vi "PRBS.vi"(7 "Fréquence \nd'echantillonage (Hz)":dbl, 8 "Entrée d'erreur\n(sans erreur)":errorcluster caption="Error in (no error)", 11 "Labview opt":T1={"Fréequence minimale (Hz)"=0.1, "Amplitude minimale (V)"=0.0, "Amplitude maximale (V)"=1.0, "Fréquence maximale (Hz)"=0.1, "Temps de simulation (min)"=2.0}) -> (0 "Sorti d'erreur":errorcluster, 2 "DSP par FFT":cluster{dbl[], dbl[]}(graph) caption="DSP approximée", 3 "u":cluster{dbl[], dbl[]}(graph))   [LabVIEW 2019]
uses:
  <vilib>/Analysis/NI_AALPro.lvlib
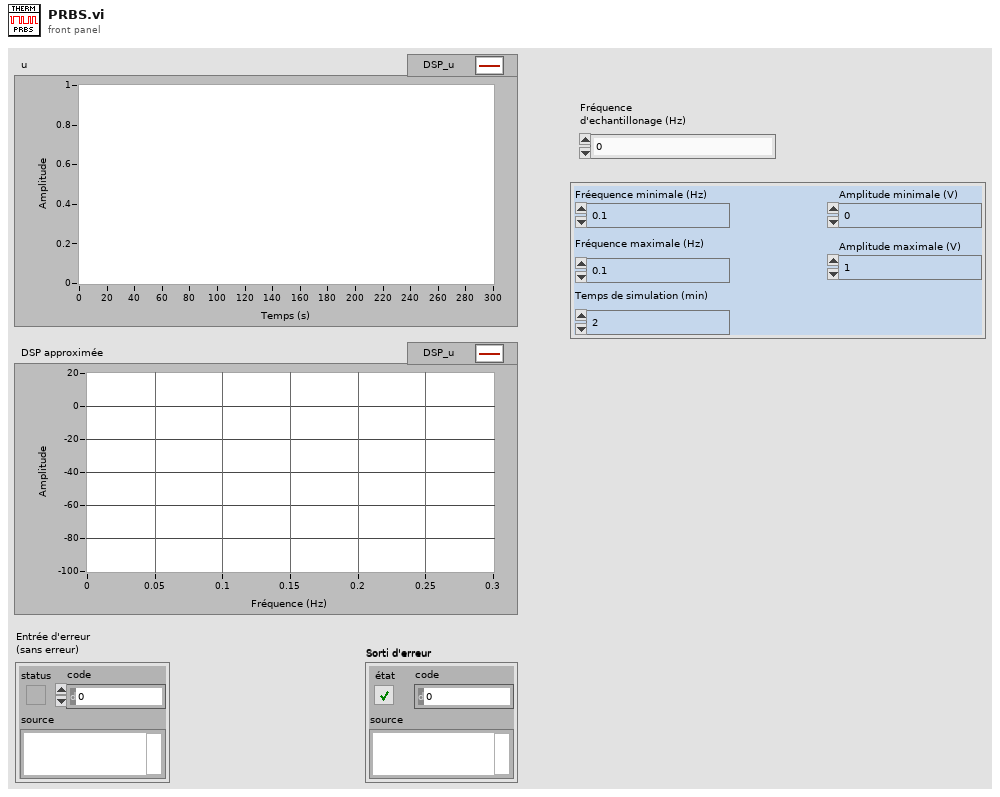
[diagram p1: front panel]
types:
  T1 = cluster{"Fréequence minimale (Hz)":dbl, "Amplitude minimale (V)":dbl, "Amplitude maximale (V)":dbl, "Fréquence maximale (Hz)":dbl, "Temps de simulation (min)":dbl}
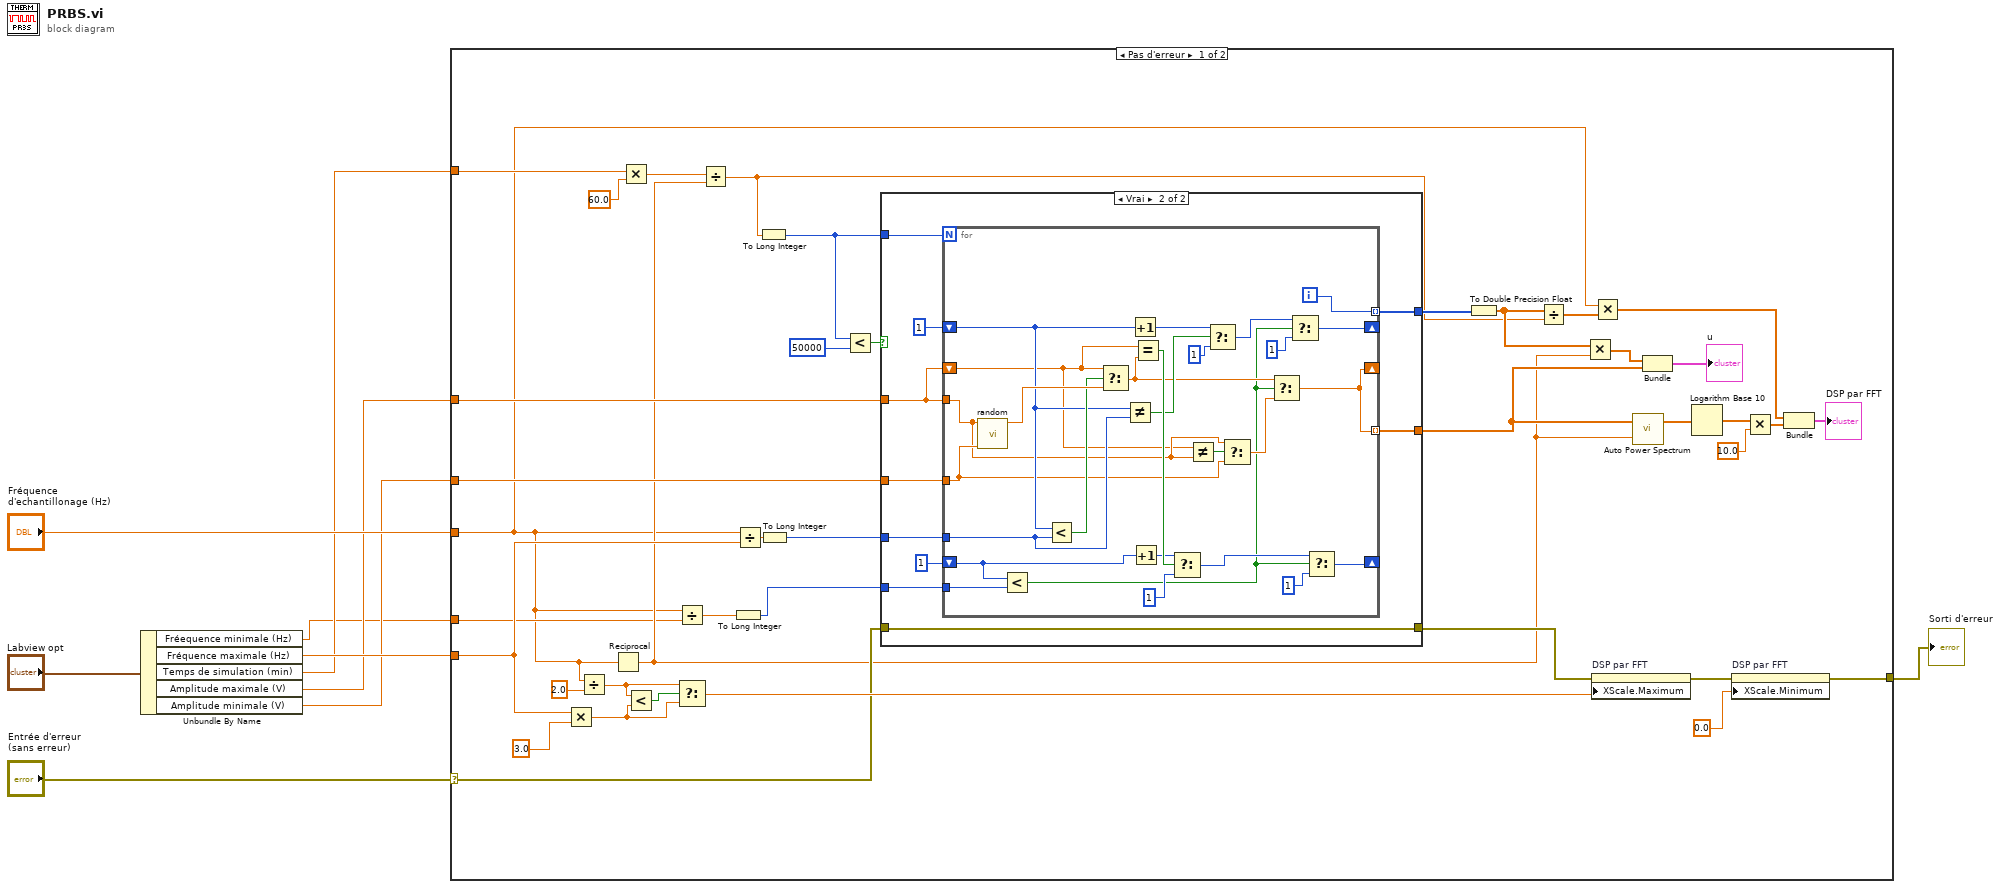
[diagram p0: block diagram]
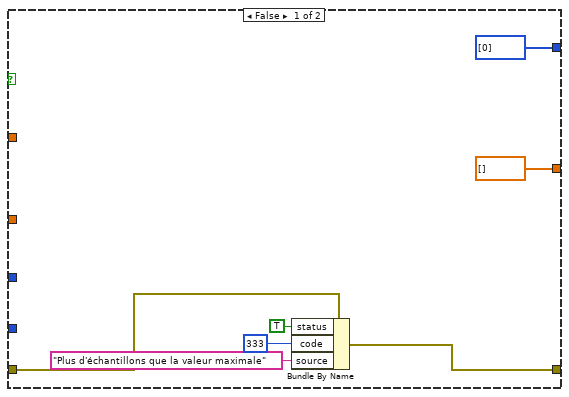
[diagram p2: hidden frame]
diagram:
  n1 = Unbundle By Name("Labview opt") -> ("Fréequence minimale (Hz)"=w1:dbl, "Fréquence maximale (Hz)"=w6:dbl, "Temps de simulation (min)"=w5:dbl, "Amplitude maximale (V)"=w3:dbl, "Amplitude minimale (V)"=w4:dbl)
  n2 = case shown="Pas d'erreur" "Entrée d'erreur\n(sans erreur)" {
    selector: "Entrée d'erreur\n(sans erreur)" -> [w16 w94]
    tunnel: "Fréquence \nd'echantillonage (Hz)" -> [w10 _]
    tunnel: w6 -> [w35 _]
    tunnel: [w27 w94] -> w7
    tunnel: w5 -> [w23 _]
    tunnel: w4 -> [w22 _]
    tunnel: w3 -> [w21 _]
    tunnel: w1 -> [w11 _]
    frame No Error {
      n3 = Multiply(x=w35, y=3.0) -> (x*y=w34:dbl)
      n4 = Divide(x=w10, y=2.0) -> (x/y=w31:dbl)
      n5 = Reciprocal(x=w10) -> (1/x=w12:dbl)
      n6 = Multiply(x=w23, y=60.0) -> (x*y=w25:dbl)
      n7 = Less?(x=w31, y=w34) -> (x < y?=w33:bool)
      n8 = Divide(x=w10, y=w11) -> (x/y=w15:dbl)
      n9 = Select(t=w31, s=w33, f=w34) -> (s? t:f=w32:dbl)
      n10 = Divide(x=w25, y=w12) -> (x/y=w29:dbl)
      n11 = To Long Integer(number=w15) -> (32bit integer=w14:i32)
      n12 = Divide(x=w10, y=w35) -> (x/y=w49:dbl)
      n13 = To Long Integer(number=w29) -> (32bit integer=w20:i32)
      n14 = To Long Integer(number=w49) -> (32bit integer=w48:i32)
      n15 = Less?(x=w20, y=50000) -> (x < y?=w19:bool)
      n16 = case shown="Vrai" w19 {
        tunnel: w48 -> [_ w66]
        tunnel: [i32[] [0] w62] -> w41
        tunnel: [dbl[] [] w59] -> w13
        tunnel: w20 -> [_ w65]
        tunnel: w22 -> [_ w64]
        tunnel: w21 -> [_ w58]
        tunnel: [w50 w63] -> w17
        tunnel: w16 -> [w54 w63]
        tunnel: w14 -> [_ w60]
        frame False {
          n17 = Bundle By Name(cluster=w54, "status"=TRUE, "code"=333, "source"="Plus d'échantillons que la valeur maximale") -> (w50:errorcluster)
        }
        frame True {
          n18 = for {
            N: w65 -> [_]
            shift-right: [w69] -> _
            shift-left: w58 -> [w67]
            tunnel: w66 -> [w77]
            tunnel: w64 -> [w74]
            tunnel: w58 -> [w71]
            shift-right: [w89] -> _
            shift-left: 1 -> [w78]
            tunnel: [w93] -> w62 mode=indexing
            tunnel: w60 -> [w90]
            tunnel: [w69] -> w59 mode=indexing
            shift-right: [w82] -> _
            shift-left: 1 -> [w75]
            i -> [w93]
            n19 = call "random.vi"("Min value"=w74, "Max value"=w71) -> ("Sortie"=w80:dbl)  [unwired: 8 in, 1 out]
            n20 = Less?(x=w75, y=w90) -> (x < y?=w68:bool)
            n21 = Less?(x=w78, y=w77) -> (x < y?=w79:bool)
            n22 = Select(t=w67, s=w79, f=w80) -> (s? t:f=w72:dbl)
            n23 = Not Equal?(x=w78, y=w77) -> (x != y?=w76:bool)
            n24 = Increment(x=w78) -> (x+1=w92:i32)
            n25 = Increment(x=w75) -> (x+1=w84:i32)
            n26 = Equal?(x=w67, y=w72) -> (x = y?=w85:bool)
            n27 = Select(t=w84, s=w85, f=1 ("cas faux")) -> (s? t:f=w81:i32)
            n28 = Not Equal?(x=w67, y=w71) -> (x != y?=w70:bool)
            n29 = Select(t=w92, s=w76, f=1 ("cas faux")) -> (s? t:f=w88:i32)
            n30 = Select(t=w71, s=w70, f=w74) -> (s? t:f=w73:dbl)
            n31 = Select(t=w72, s=w68, f=w73) -> (s? t:f=w69:dbl)
            n32 = Select(t=w88, s=w68, f=1 ("cas faux")) -> (s? t:f=w89:i32)
            n33 = Select(t=w81, s=w68, f=1 ("cas faux")) -> (s? t:f=w82:i32)
          }
        }
      }
      n34 = To Double Precision Float(number=w41) -> (double precision float=w36:dbl[])
      n35 = Divide(x=w36, y=w29) -> (x/y=w40:dbl[])
      n36 = Multiply(x=w36, y=w12) -> (x*y=w37:dbl[])
      n37 = property on="DSP par FFT" class="GraphXY (strict)"(error in=w17, "XScale.Maximum"=w32) -> (error out=w28:errorcluster)  [unwired: 1 in, 1 out]
      n38 = Multiply(x=w10, y=w40) -> (x*y=w39:dbl[])
      n39 = call <vilib>:"Auto Power Spectrum.vi"("dt"=w12, "Signal (V)"=w13) -> ("Power Spectrum (V^2 rms)"=w47:dbl[])  [unwired: 1 out]
      n40 = Bundle(w37, w13) -> (→"u":cluster{dbl[], dbl[]})  [unwired: 1 in]
      n41 = Logarithm Base 10(1:w47) -> (0:w46:dbl[])
      n42 = property on="DSP par FFT" class="GraphXY (strict)"(error in=w28, "XScale.Minimum"=0.0 ("Échelle des X.Gamme:Minimum")) -> (error out=w27:errorcluster)  [unwired: 1 in, 1 out]
      n43 = Multiply(x=w46, y=10.0 ("x")) -> (x*y=w42:dbl[])
      n44 = Bundle(w39, w42) -> (→"DSP par FFT":cluster{dbl[], dbl[]})  [unwired: 1 in]
    }
    frame Error {
    }
  }
  "Sorti d'erreur" <- w7
